vi "Przeładowanie punktu startowego i punktów docelowych.vi"(6 "Pocz. poł. in":T3, 9 "Lista współrzędnych":string[][](array[string]), 10 "Właściwości mapy":T2, 11 "Mapa terenu":picture) -> (3 "Mapa z wprowadzonym punktem":picture)   [LabVIEW 2012, in "Biblioteka moduł map v3.lvlib" / "Obsługa grafiki mapy.lvlib"]
uses:
  <vilib>/Utility/miscctls.llb/LVBoundsTypeDef.ctl
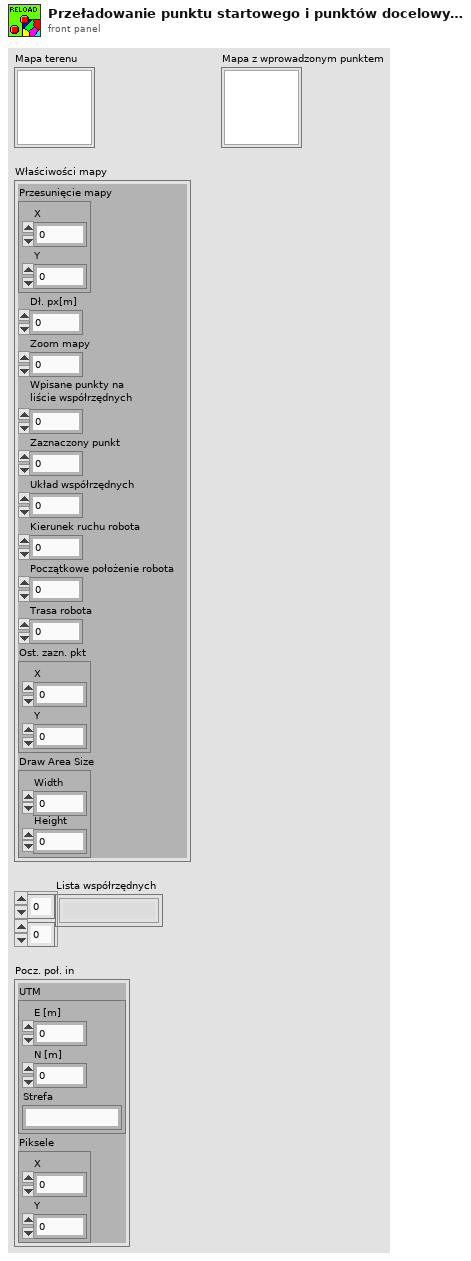
[diagram p1: front panel]
types:
  T1 = typedef "LVBoundsTypeDef.ctl" = cluster{"Width":u32, "Height":u32}
  T2 = cluster{"Przesunięcie mapy":cluster{"X":i16, "Y":i16}, "Dł. px[m]":dbl, "Zoom mapy":sgl, "Wpisane punkty na\nliście współrzędnych":u32, "Zaznaczony punkt":u32, "Układ współrzędnych":u32, "Kierunek ruchu robota":u32, "Początkowe położenie robota":u32, "Trasa robota":u32, "Ost. zazn. pkt":cluster{"X":i32, "Y":i32}, "Draw Area Size":T1}
  T3 = cluster{"UTM":cluster{"E [m]":ext, "N [m]":ext, "Strefa":string}, "Piksele":cluster{"X":i32, "Y":i32}}
  T4 = cluster{"Kolor punktów z listy":u32, "Położenie startowe robota":cluster{"Pixel y":i16, "Pixel x":i16}}
  T5 = cluster{"Położenie":cluster{"Pixel x":i16, "Pixel y":i16}, "Kolor punktu":u32, "Rozmiar punktu":u32, "Nazwa punktu":string}
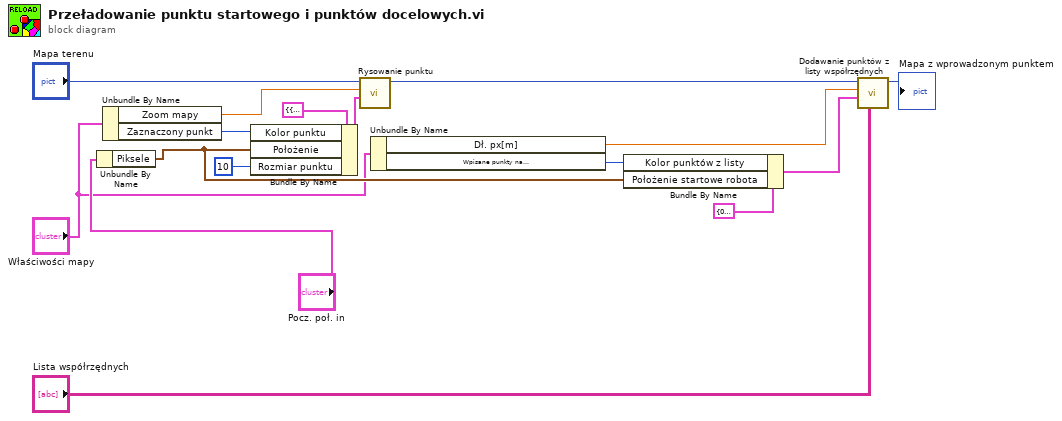
[diagram p0: block diagram]
diagram:
  n1 = Unbundle By Name("Pocz. poł. in") -> ("Piksele"=w13:cluster{"X":i32, "Y":i32})
  n2 = Unbundle By Name("Właściwości mapy") -> ("Zoom mapy"=w5:sgl, "Zaznaczony punkt"=w6:u32)
  n3 = Bundle By Name(cluster=T5 {"Położenie"={"Pixel x"=246, "Pixel y"=243}, "Kolor punktu"=15663118, "Rozmiar punktu"=2, "Nazwa punktu"="START"} ("Punkt na mapie"), "Kolor punktu"=w6, "Położenie"=w13, "Rozmiar punktu"=u32 10) -> (w4:T5)
  n4 = call "Rysowanie punktu.vi"("Punkt na mapie"=w4, "Zoom mapy"=w5, "Mapa terenu"="Mapa terenu") -> ("Mapa z wprowadzonym punktem"=w10:picture)  [unwired: 8 in]
  n5 = Unbundle By Name("Właściwości mapy") -> ("Dł. px[m]"=w8:dbl, "Wpisane punkty na\nliście współrzędnych"=w7:u32)
  n6 = Bundle By Name(cluster=T4 {"Kolor punktów z listy"=0, "Położenie startowe robota"={"Pixel y"=0, "Pixel x"=0}} ("Właściwości punktów z listy"), "Kolor punktów z listy"=w7, "Położenie startowe robota"=w13) -> (w9:T4)
  n7 = call "Dodawanie punktów z listy współrzędnych.vi"("Lista współrzędnych"="Lista współrzędnych", "Właściwości punktów z listy"=w9, "Długość piksela w metrach"=w8, "Mapa terenu"=w10) -> ("Mapa z wprowadzonym punktem"=→"Mapa z wprowadzonym punktem":picture)  [unwired: 6 in, 1 out]
